vi "To JSON.vi"(8 "error in (no error)":errorcluster, 11 "Configuration Base in":refnum<class "Config Base.lvclass">) -> (0 "error out":errorcluster, 3 "Configuration Base out":refnum<class "Config Base.lvclass">)   [LabVIEW 2023, in "HAL GOOP4.lvlib" / "Config Base.lvclass"]
uses:
  Config Base.lvclass
  Config Base.lvclass/Config Base.ctl
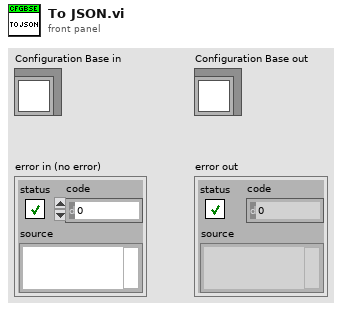
[diagram p1: front panel]
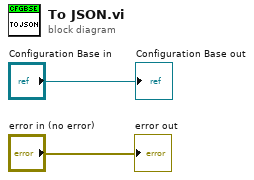
[diagram p0: block diagram]
diagram:
  "error out" <- "error in (no error)"
  "Configuration Base out" <- "Configuration Base in"
